vi "control lazer.vi"(9 "last timer value":u32, 10 "able to shoot _1":bool) -> (3 "timer value":u32)   [LabVIEW 2012]
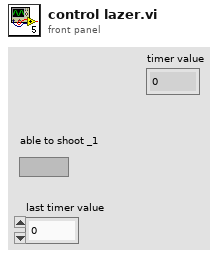
[diagram p1: front panel]
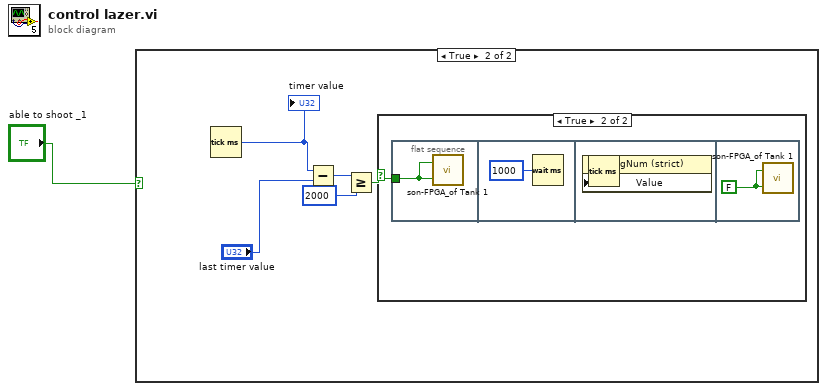
[diagram p0: block diagram]
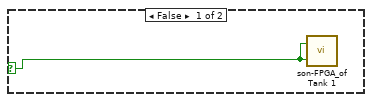
[diagram p2: hidden frame]
diagram:
  n1 = case shown="True" "able to shoot _1" {
    selector: "able to shoot _1" -> [w2 _]
    frame False {
      n2 = call "son-FPGA_of Tank 1.vi"("Port9/DIO8"=w2, "stop"=w2) -> ()  [unwired: 1 in]
    }
    frame True {
      n3 = Tick Count (ms)() -> (millisecond timer value=w7:u32)
      "timer value" <- w7
      n4 = Subtract(x=w7, y="last timer value") -> (x-y=w5:u32)
      n5 = Greater Or Equal?(x=w5, y=u32 2000) -> (x >= y?=w3:bool)
      n6 = case shown="True" w3 {
        selector: w3 -> [_ w8]
        frame False {
        }
        frame True {
          n7 = flat-sequence {
            tunnel: w8 -> [w9]
            frame #0 {
              n8 = call "son-FPGA_of Tank 1.vi"("Port9/DIO8"=w9, "stop"=w9) -> ()  [unwired: 1 in]
            }
            frame #1 {
              n9 = Wait (ms)(milliseconds to wait=u32 1000) -> ()  [unwired: 1 out]
            }
            frame #2 {
              n10 = Tick Count (ms)() -> (millisecond timer value=w11:u32)
              n11 = property class="DigNum (strict)"("Value"=w11) -> ()  [unwired: 2 in, 2 out]
            }
            frame #3 {
              w12 = FALSE ("Port9/DIO8")
              n12 = call "son-FPGA_of Tank 1.vi"("Port9/DIO8"=w12, "stop"=w12) -> ()  [unwired: 1 in]
            }
          }
        }
      }
    }
  }
